vi "get_amp_phas.vi"(8 "error in (no error)":errorcluster, 11 "SR 830 & NI USB7855R in":refnum<class "SR 830 & NI USB7855R.lvclass">) -> (0 "error out":errorcluster, 1 "Phase (rad)":dbl, 2 "Amplitude (V rms)":dbl, 3 "SR 830 & NI USB7855R out":refnum<class "SR 830 & NI USB7855R.lvclass">)   [LabVIEW 2020, in "SR 830 & NI USB7855R.lvclass"]
uses:
  SR 830 & NI USB7855R.lvclass
  SR 830 & NI USB7855R.lvclass/SR 830 & NI USB7855R.ctl
  <vilib>/Utility/error.llb/Error Cluster From Error Code.vi
  <vilib>/rvi/errors/niLvFpgaAdjustHostInterfaceError.vi
  <vilib>/rvi/interface/nirviReadWriteControl/nirviReadWriteControl.xnode
  NiFpgaLv.dll
  <vilib>/rvi/interface/Simulation/niFpgaSimulationCallBeginRW.vi
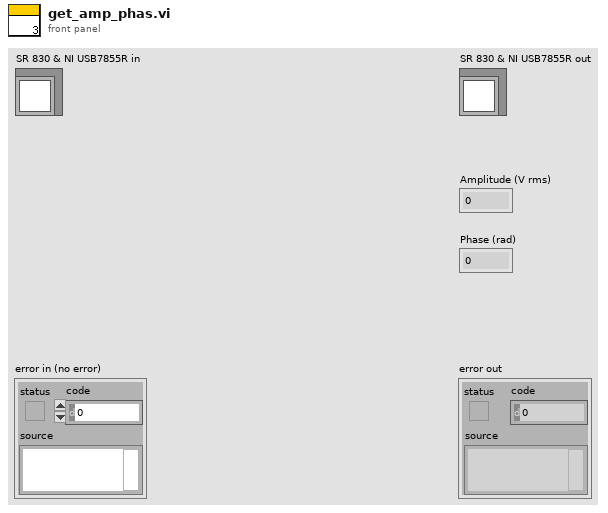
[diagram p1: front panel]
types:
  T1 = enum16{"USB 7855 (AI)", "USB 7855 (AO)", "USB 7855 OEM (AI)", "USB 7855 OEM (AO)", "USB 7856  (AI)", "USB 7856 (AO)", "USB 7856 OEM (AI)", "USB 7856 OEM (AO)"}
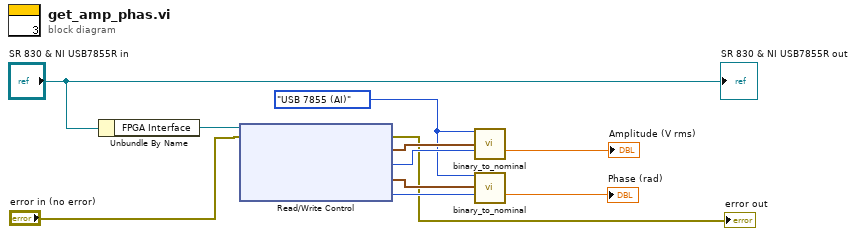
[diagram p0: block diagram]
diagram:
  w5 = T1."USB 7855 (AI)" ("Target Type")
  n1 = Unbundle By Name("SR 830 & NI USB7855R in") -> ("FPGA Interface"=w11:refnum<k20>)
  n2 = xnode "Read/Write Control"("FPGA VI Reference In"=w11, "error in"="error in (no error)") -> ("error out"=→"error out":errorcluster, "AI2 Calibration Constants"=w9:cluster{u32, i32}, "Lock-in Amplitude"=w8:i16, "AI3 Calibration Constants"=w7:cluster{u32, i32}, "Lock-in Phase"=w6:i16)  [unwired: 1 out]
  n3 = call "binary_to_nominal.vi"("Target Type"=w5, "Channel Calibration"=w9, "Binary Value"=w8) -> ("Nominal Value"=→"Amplitude (V rms)":dbl)  [unwired: 11 in, 1 out]
  n4 = call "binary_to_nominal.vi"("Target Type"=w5, "Channel Calibration"=w7, "Binary Value"=w6) -> ("Nominal Value"=→"Phase (rad)":dbl)  [unwired: 11 in, 1 out]
  "SR 830 & NI USB7855R out" <- "SR 830 & NI USB7855R in"
